vi "Information.vi"(8 "error in (no error)":errorcluster, 9 "Context":T1, 10 "Information":refnum<class "Information.lvclass">, 11 "Pulse Controller in":refnum<class "Pulse Controller.lvclass">) -> (0 "error out":errorcluster, 3 "Pulse Controller out":refnum<class "Pulse Controller.lvclass">)   [LabVIEW 2021, in "Pulse Controller.lvclass"]
uses:
  Pulse Controller.lvclass
  Publish-Subscribe/Interfaces/Information/Information.lvclass
  Publish-Subscribe/Context.ctl
  Process Controller/Process Controller.lvclass
  Pulse Controller.lvclass/Pulse Controller.ctl
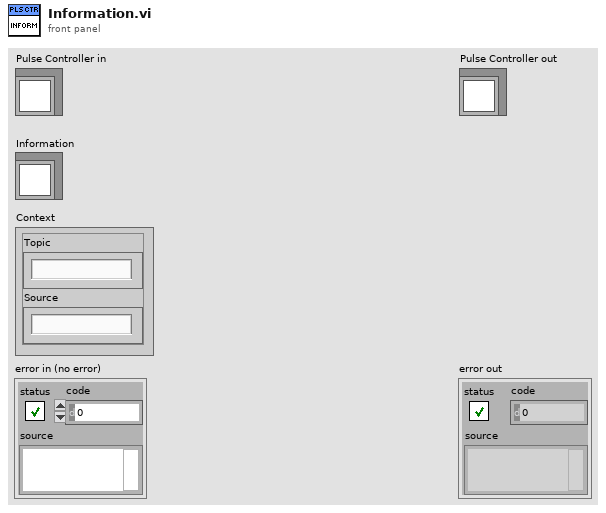
[diagram p1: front panel]
types:
  T1 = typedef "Context.ctl" = cluster{"Topic":string, "Source":string}
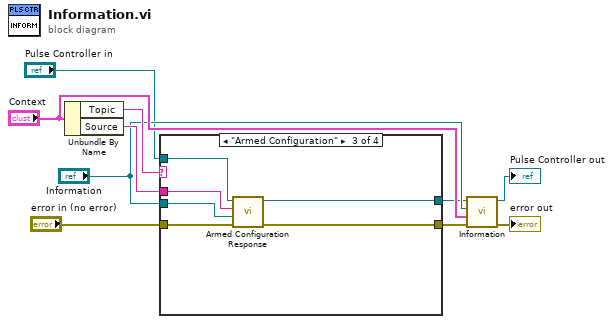
[diagram p0: block diagram]
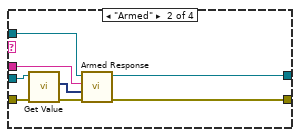
[diagram p3: hidden frame]
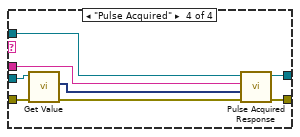
[diagram p4: hidden frame]
diagram:
  n1 = Unbundle By Name("Context") -> ("Topic"=w9:string, "Source"=w8:string)
  n2 = case shown="\"Armed Configuration\"" w9 {
    tunnel: w8 -> [_ w20 w22 w32]
    tunnel: "error in (no error)" -> [w11 w16 w23 w33]
    tunnel: "Pulse Controller in" -> [w12 w19 w26 w30]
    tunnel: "Information" -> [_ w18 w21 w34]
    tunnel: [w11 w14 w25 w27] -> w4
    tunnel: [w12 w13 w24 w29] -> w5
    frame "", Default {
    }
    frame "Armed" {
      n3 = call-dynamic "Get Value.vi"("error in (no error)"=w16, "Information in"=w18) -> ("error out"=w15:errorcluster, "Value"=w17:dynamicdata)  [unwired: 7 in, 1 out]
      n4 = call-dynamic "Armed Response.vi"("error in (no error)"=w15, "Armed"=w17, "Sender"=w20, "Pulse Controller in"=w19) -> ("error out"=w14:errorcluster, "Pulse Controller out"=w13:refnum<class "Pulse Controller.lvclass">)  [unwired: 6 in]
    }
    frame "Armed Configuration" {
      n5 = call-dynamic "Armed Configuration Response.vi"("error in (no error)"=w23, "Information"=w21, "Sender"=w22, "Pulse Controller in"=w26) -> ("error out"=w25:errorcluster, "Pulse Controller out"=w24:refnum<class "Pulse Controller.lvclass">)  [unwired: 6 in]
    }
    frame "Pulse Acquired" {
      n6 = call-dynamic "Get Value.vi"("error in (no error)"=w33, "Information in"=w34) -> ("error out"=w28:errorcluster, "Value"=w31:dynamicdata)  [unwired: 7 in, 1 out]
      n7 = call-dynamic "Pulse Acquired Response.vi"("error in (no error)"=w28, "Acquired"=w31, "Sender"=w32, "Pulse Controller in"=w30) -> ("error out"=w27:errorcluster, "Pulse Controller out"=w29:refnum<class "Pulse Controller.lvclass">)  [unwired: 6 in]
    }
  }
  n8 = call-parent "Information.vi"("error in (no error)"=w4, "Context"="Context", "Information"="Information", "Process Controller in"=w5) -> ("error out"=→"error out":errorcluster, "Process Controller out"=→"Pulse Controller out":refnum<class "Pulse Controller.lvclass">)  [unwired: 6 in]
